vi "Joystick.vi"() -> ()   [LabVIEW 2020]
uses:
  <vilib>/Rock Robotics/WPI/Utilities/WPI_GetSetVariantRefNum.vi
  GlobalVariables.vi
  <vilib>/Rock Robotics/Network Tables/NT Write Number.vi
  <vilib>/Rock Robotics/WPI/RobotDrive/WPI_RobotDriveArcadeDrive_Standard(NoSaturation).vi
  <vilib>/Rock Robotics/WPI/ThirdParty/Phoenix-LabVIEW/Motor Controller/Controls/CTRE_Phoenix_MotorControl_ControlMode.ctl
panel:
  out "Hori":dbl
  out "Vert":dbl
  out "L_X":dbl
  out "L_Y":dbl
  out "Axes[3]":dbl
  out "Axes[2]":dbl
  out "Motor Values":dbl[](array[numeric])
  out "Axes[1]":dbl
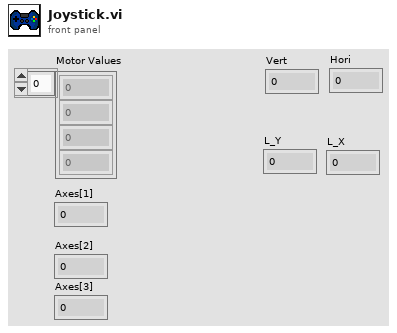
[diagram p1: front panel]
types:
  T1 = cluster{"Axes[0]":dbl, "Axes[1]":dbl, "Axes[2]":dbl, "Axes[3]":dbl, "Axes[4]":dbl, "Axes[5]":dbl, "Axes[6]":dbl, "Axes[7]":dbl, "Axes[8]":dbl}
  T2 = cluster{"Buttons[0]":bool, "Buttons[1]":bool, "Buttons[2]":bool, "Buttons[3]":bool, "Buttons[4]":bool, "Buttons[5]":bool, "Buttons[6]":bool, "Buttons[7]":bool, "Buttons[8]":bool, "Buttons[9]":bool}
  T3 = typedef "WPI_RobotDriveDevRef.ctl" = cluster{"DevStatus":errorcluster, "Motors[]":T4[], "Square Inputs":bool, "Max Output":dbl}
  T4 = typedef "WPI_MotorControlDeviceRef.ctl" = cluster{"DeviceStatus":errorcluster, "Type":T5, "PWM":cluster{"PWM Channel":T6, "DeadBand":T7}, "CAN":cluster{"Device Number":u8, "SetOutput VI Ref":variant, "GetOutput VI Ref":variant, "Enable VI Ref":variant, "Disable VI Ref":variant, "Data":variant}, "Invert":bool, "DIO PWM":cluster{"PWM \"Enable\" Channel":T6, "DIOChannel":T8, "PWM Rate":dbl}}
  T5 = typedef "WPI_MotorControlType.ctl" = enum16{"PWM", "CAN", "DIO PWM"}
  T6 = typedef "FPGA_DIOPWMChannel.ctl" = enum8{"PWM 0", "PWM 1", "PWM 2", "PWM 3", "PWM 4", "PWM 5", "PWM 6", "PWM 7", "PWM 8", "PWM 9", "PWM MXP 0", "PWM MXP 1", "PWM MXP 2", "PWM MXP 3", "PWM MXP 4", "PWM MXP 5", "PWM MXP 6", "PWM MXP 7", "PWM MXP 8", "PWM MXP 9", "Invalid"}
  T7 = typedef "WPI_PWMDeadband.ctl" = cluster{"Name":string, "maxPositivePwm":i32, "minPositivePwm":i32, "centerPwm":i32, "maxNegativePwm":i32, "minNegativePwm":i32, "angularRange":u16}
  T8 = typedef "FPGA_DIOChannel.ctl" = enum8{"DIO 0", "DIO 1", "DIO 2", "DIO 3", "DIO 4", "DIO 5", "DIO 6", "DIO 7", "DIO 8", "DIO 9", "DIO MXP 0", "DIO MXP 1", "DIO MXP 2", "DIO MXP 3", "DIO MXP 4", "DIO MXP 5", "DIO MXP 6", "DIO MXP 7", "DIO MXP 8", "DIO MXP 9", "DIO MXP 10", "DIO MXP 11", "DIO MXP 12", "DIO MXP 13", "DIO MXP 14", "DIO MXP 15", "SPI Port CS1", "SPI Port CS2", "SPI Port CS3", "SPI Port MISO", "SPI Port MOSI", "Invalid"}
  T9 = typedef "CTRE_Phoenix_MotorControl_ControlMode.ctl" = u16
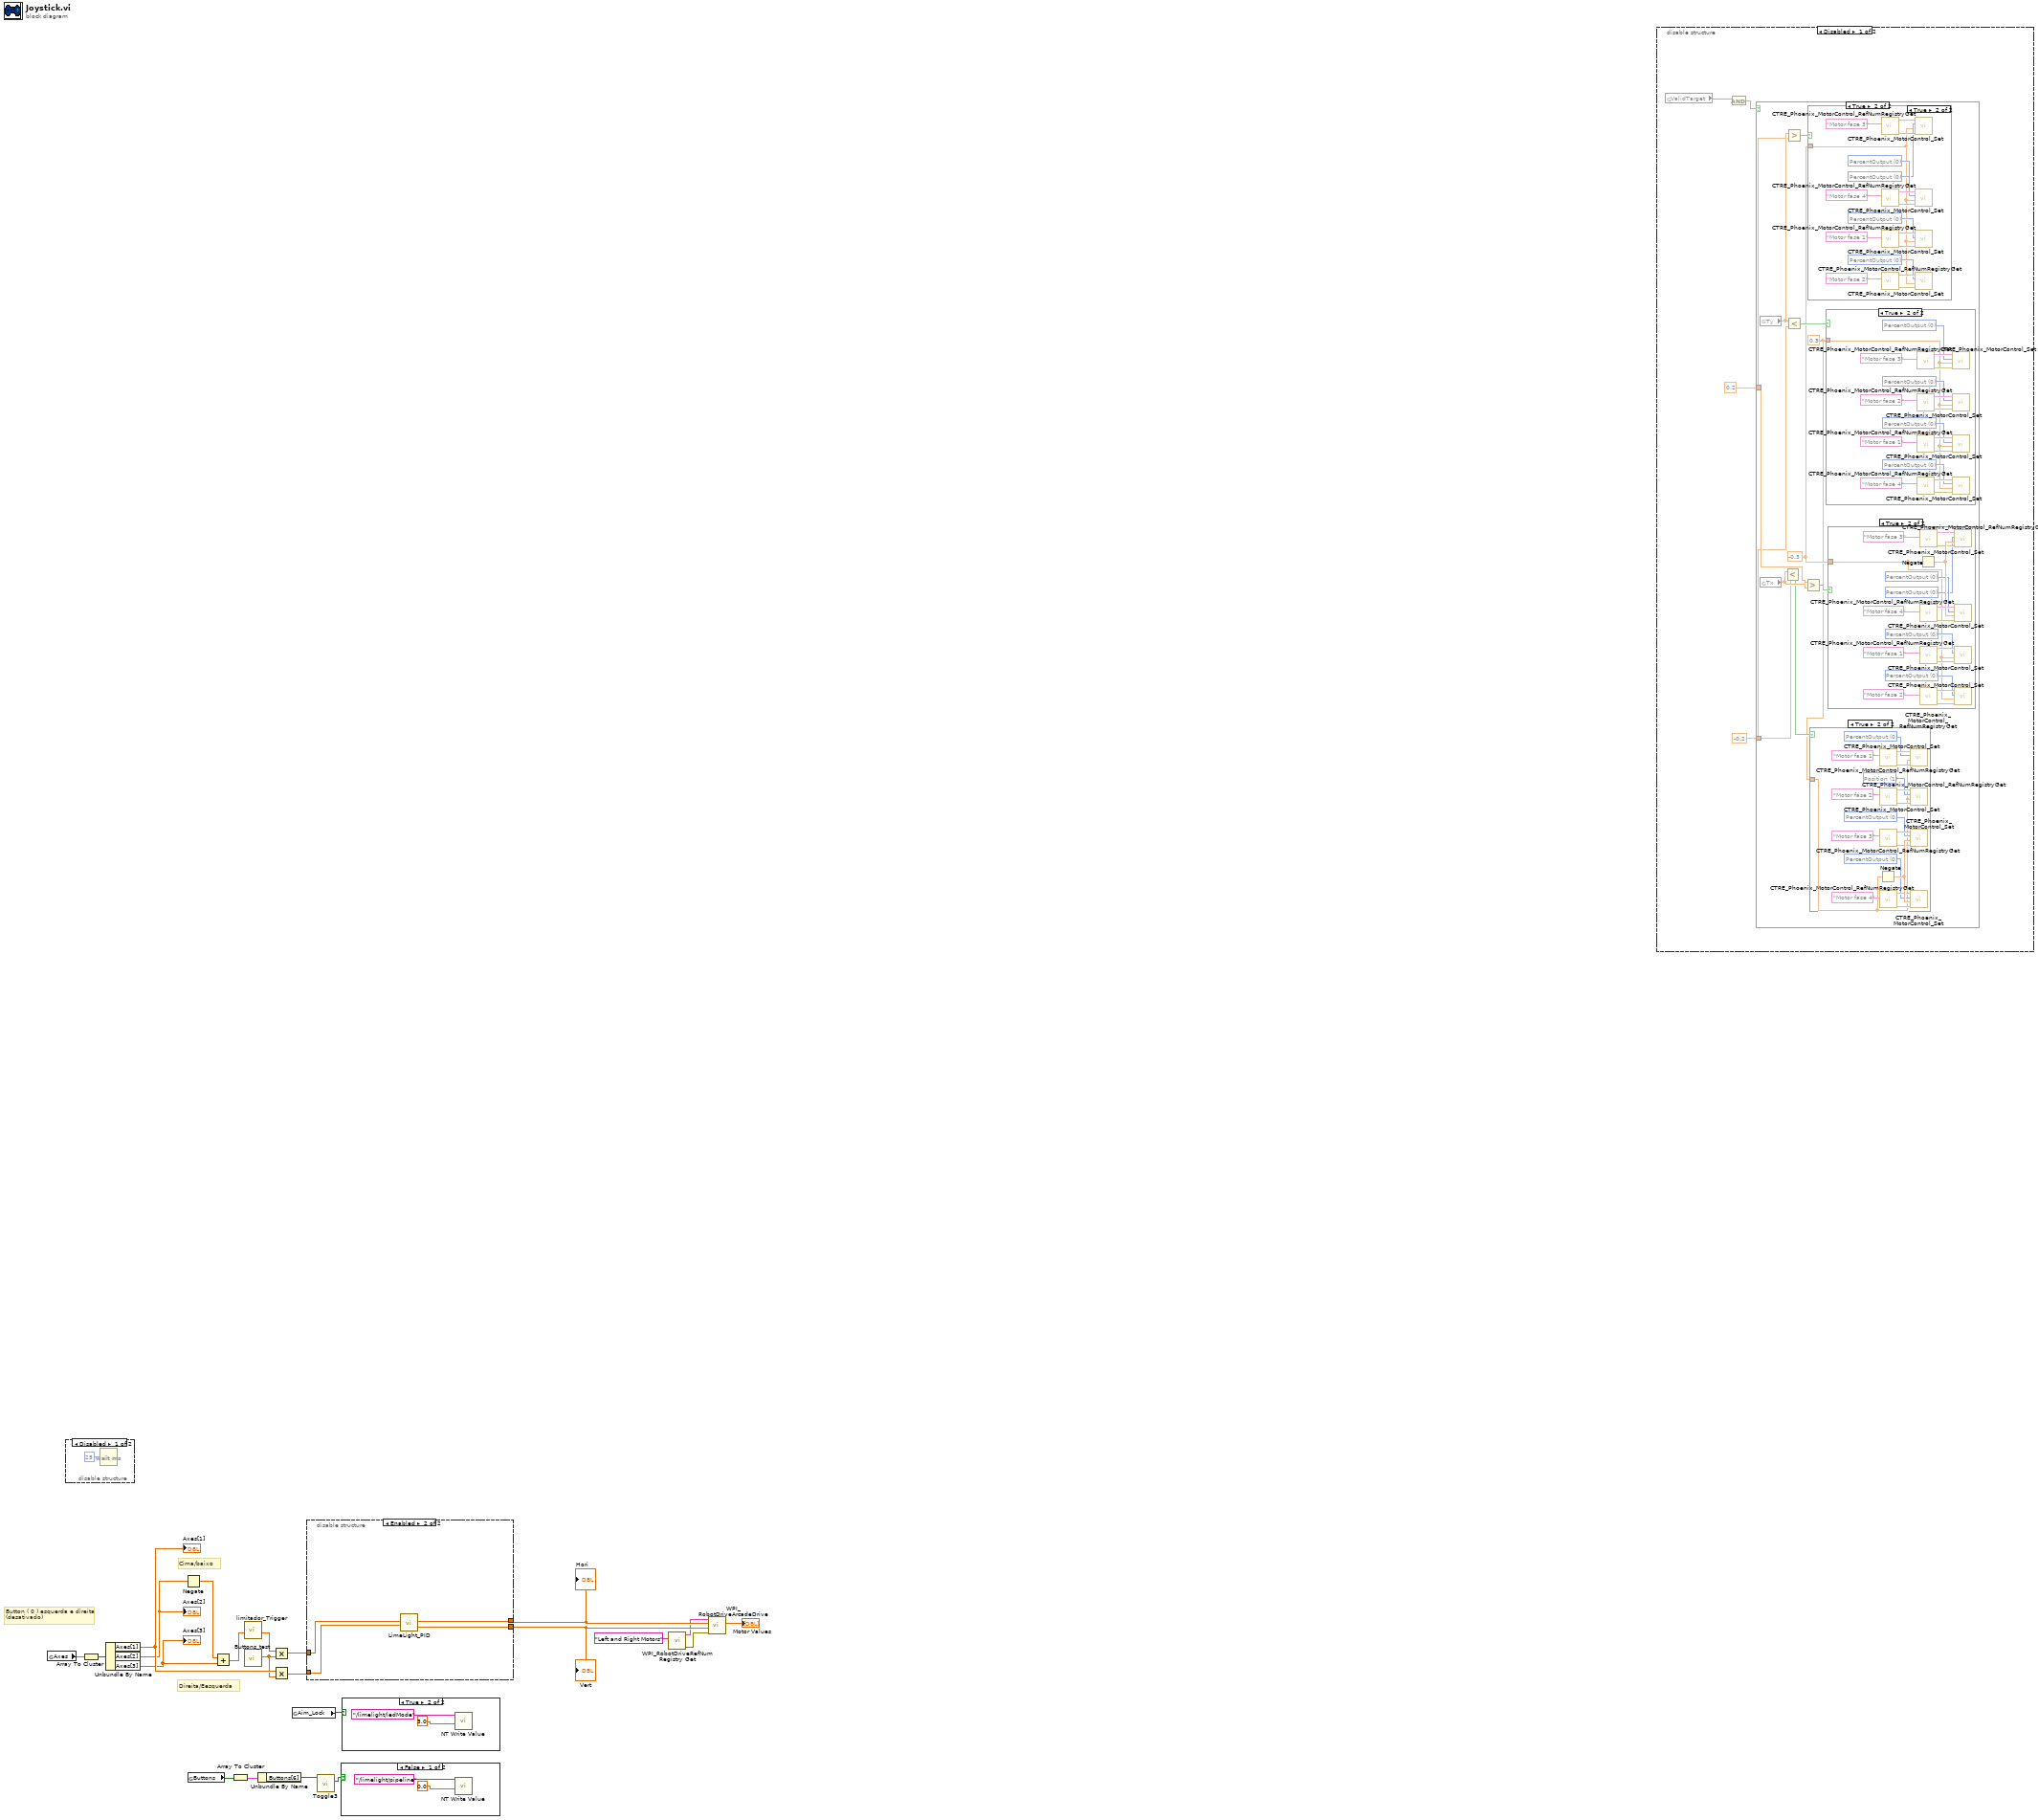
[diagram p0: block diagram]
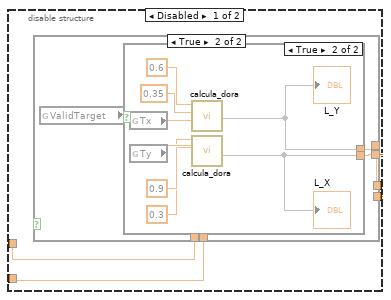
[diagram p3: hidden frame]
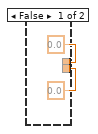
[diagram p5: hidden frame]
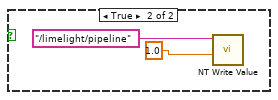
[diagram p6: hidden frame]
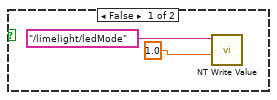
[diagram p7: hidden frame]
diagram:
  # "Button ( 0 ) esquerda e direita \n(desativado)"
  # "Direita/Eesquerda"
  # "Cima/baixo"
  n1 = global read "GlobalVariables.vi" "Axes"() -> (w3:dbl[])
  n2 = disable-structure shown="Disabled" {
    frame Disabled {
      n3 = Wait (ms)(milliseconds to wait=u32 25) -> ()  [unwired: 1 out]
    }
    frame Enabled {
    }
  }
  n4 = Array To Cluster(array=w3) -> (cluster=w4:T1)
  n5 = Unbundle By Name(w4) -> ("Axes[1]"=w22:dbl, "Axes[2]"=w18:dbl, "Axes[3]"=w7:dbl)
  "Axes[1]" <- w22
  "Axes[2]" <- w18
  "Axes[3]" <- w7
  n6 = Negate(x=w18) -> (-x=w17:dbl)
  n7 = global read "GlobalVariables.vi" "Buttons"() -> (w5:bool[])
  n8 = Add(x=w17, y=w7) -> (x+y=w20:dbl)
  n9 = Array To Cluster(array=w5) -> (cluster=w6:T2)
  n10 = call "limitador_Trigger.vi"("IN"=w20) -> ("OUT"=w19:dbl)  [unwired: 10 in]
  n11 = call "Buttons_test.vi"() -> ("OUT"=w21:dbl)  [unwired: 9 in]
  n12 = Unbundle By Name(w6) -> ("Buttons[6]"=w1:bool)
  n13 = Multiply(x=w19, y=w21) -> (x*y=w15:dbl)
  n14 = Multiply(x=w22, y=w21) -> (x*y=w16:dbl)
  n15 = global read "GlobalVariables.vi" "Aim_Lock"() -> (w8:bool)
  n16 = disable-structure shown="Enabled" {
    disable-tunnel: w16 -> [w27 w44]
    disable-tunnel: w15 -> [w26 w46]
    disable-tunnel: [w25 w45] -> w14
    disable-tunnel: [w24 w43] -> w13
    frame Disabled {
      n17 = case shown="True" {
        selector: _ -> [_ _]
        tunnel: w27 -> [w29 _]
        tunnel: w26 -> [w28 _]
        tunnel: [w29 w31] -> w25
        tunnel: [w28 w32] -> w24
        frame False {
        }
        frame True {
          n18 = global read "GlobalVariables.vi" "ValidTarget"() -> (w30:bool)
          n19 = case shown="True" w30 {
            tunnel: [0.0 ("x+y") w42] -> w32
            tunnel: [0.0 ("x+y") w39] -> w31
            frame False {
            }
            frame True {
              n20 = global read "GlobalVariables.vi" "Tx"() -> (w41:dbl)
              n21 = global read "GlobalVariables.vi" "Ty"() -> (w40:dbl)
              n22 = call "calcula_dora.vi"(9:w41, 10:0.35, 11:0.6) -> (1:w42)  [unwired: 8 in]
              "L_Y" <- w42
              n23 = call "calcula_dora.vi"(9:w40, 10:0.3, 11:0.9) -> (1:w39)  [unwired: 8 in]
              "L_X" <- w39
            }
          }
        }
      }
    }
    frame Enabled {
      n24 = call "LimeLight_PID.vi"("Numeric 2"=w44, "Numeric"=w46) -> ("output_ty"=w45:dbl, "output_tx"=w43:dbl)  [unwired: 8 in]
    }
  }
  "Vert" <- w14
  "Hori" <- w13
  n25 = call "Toggle3.vi"("Input3"=w1) -> ("Output3"=w2:bool)  [unwired: 10 in]
  n26 = case shown="False" w2 {
    frame False {
      n27 = call-poly <vilib>:"NT Write Value.vi"("Numeric"=0.0, "Name"="/limelight/pipeline") -> ()  [unwired: 9 in, 1 out]
    }
    frame True {
      n28 = call-poly <vilib>:"NT Write Value.vi"("Numeric"=1.0, "Name"="/limelight/pipeline") -> ()  [unwired: 9 in, 1 out]
    }
  }
  n29 = case shown="True" w8 {
    frame False {
      n30 = call-poly <vilib>:"NT Write Value.vi"("Numeric"=1.0, "Name"="/limelight/ledMode") -> ()  [unwired: 9 in, 1 out]
    }
    frame True {
      n31 = call-poly <vilib>:"NT Write Value.vi"("Numeric"=3.0, "Name"="/limelight/ledMode") -> ()  [unwired: 9 in, 1 out]
    }
  }
  n32 = call <vilib>:"WPI_RobotDriveRefNum Registry Get.vi"("refnum name"="Left and Right Motors") -> ("error out"=w9:errorcluster, "RobotDriveDevRef"=w11:T3)  [unwired: 9 in]
  n33 = call-poly <vilib>:"WPI_RobotDriveArcadeDrive.vi"("error in (no error)"=w9, "Y axis value"=w14, "X axis value"=w13, "RobotDriveDevRef"=w11) -> ("Motor Values"=→"Motor Values":dbl[])  [unwired: 5 in, 2 out]
  n34 = disable-structure shown="Disabled" {
    frame Disabled {
      n35 = global read "GlobalVariables.vi" "ValidTarget"() -> (w58:bool)
      n36 = And(x=w58) -> (x .and. y?=w57:bool)  [unwired: 1 in]
      n37 = case shown="True" w57 {
        tunnel: 0.2 -> [_ w62]
        tunnel: -0.2 -> [_ w61]
        frame False {
        }
        frame True {
          w59 = 0.3
          w60 = -0.3
          n38 = global read "GlobalVariables.vi" "Ty"() -> (w64:dbl)
          n39 = global read "GlobalVariables.vi" "Tx"() -> (w67:dbl)
          n40 = Less?(x=w67, y=w61) -> (x < y?=w66:bool)
          n41 = Greater?(x=w64, y=w62) -> (0:w65:bool)
          n42 = Less?(x=w64, y=w61) -> (x < y?=w63:bool)
          n43 = Greater?(x=w67, y=w62) -> (0:w68:bool)
          n44 = case shown="True" w65 {
            tunnel: w60 -> [_ w86]
            frame False {
            }
            frame True {
              w94 = T9 0 items=["PercentOutput"=0, "Position"=1, "Velocity"=2, "Current"=3, "Follower"=5, "MotionProfile"=6, "MotionMagic"=7, "MotionProfileArc"=10, "Disabled"=15] ("Control Mode")
              w92 = T9 0 items=["PercentOutput"=0, "Position"=1, "Velocity"=2, "Current"=3, "Follower"=5, "MotionProfile"=6, "MotionMagic"=7, "MotionProfileArc"=10, "Disabled"=15] ("Control Mode")
              w90 = T9 0 items=["PercentOutput"=0, "Position"=1, "Velocity"=2, "Current"=3, "Follower"=5, "MotionProfile"=6, "MotionMagic"=7, "MotionProfileArc"=10, "Disabled"=15] ("Control Mode")
              w88 = T9 0 items=["PercentOutput"=0, "Position"=1, "Velocity"=2, "Current"=3, "Follower"=5, "MotionProfile"=6, "MotionMagic"=7, "MotionProfileArc"=10, "Disabled"=15] ("Control Mode")
              n45 = call <vilib>:"CTRE_Phoenix_MotorControl_RefNumRegistryGet.vi"("refnum name"="Motor fase 3") -> ("error out"=w96:errorcluster, "PhoenixMotorControlDevRef"=w95:T4)  [unwired: 9 in]
              n46 = call <vilib>:"CTRE_Phoenix_MotorControl_RefNumRegistryGet.vi"("refnum name"="Motor fase 4") -> ("error out"=w98:errorcluster, "PhoenixMotorControlDevRef"=w97:T4)  [unwired: 9 in]
              n47 = call <vilib>:"CTRE_Phoenix_MotorControl_RefNumRegistryGet.vi"("refnum name"="Motor fase 1") -> ("error out"=w100:errorcluster, "PhoenixMotorControlDevRef"=w99:T4)  [unwired: 9 in]
              n48 = call <vilib>:"CTRE_Phoenix_MotorControl_RefNumRegistryGet.vi"("refnum name"="Motor fase 2") -> ("error out"=w102:errorcluster, "PhoenixMotorControlDevRef"=w101:T4)  [unwired: 9 in]
              n49 = call <vilib>:"CTRE_Phoenix_MotorControl_Set.vi"("error in (no error)"=w96, "Output"=w86, "Control Mode"=w88, "PhoenixMotorControlDevRef"=w95) -> ()  [unwired: 6 in, 2 out]
              n50 = call <vilib>:"CTRE_Phoenix_MotorControl_Set.vi"("error in (no error)"=w98, "Output"=w86, "Control Mode"=w90, "PhoenixMotorControlDevRef"=w97) -> ()  [unwired: 6 in, 2 out]
              n51 = call <vilib>:"CTRE_Phoenix_MotorControl_Set.vi"("error in (no error)"=w100, "Output"=w86, "Control Mode"=w92, "PhoenixMotorControlDevRef"=w99) -> ()  [unwired: 6 in, 2 out]
              n52 = call <vilib>:"CTRE_Phoenix_MotorControl_Set.vi"("error in (no error)"=w102, "Output"=w86, "Control Mode"=w94, "PhoenixMotorControlDevRef"=w101) -> ()  [unwired: 6 in, 2 out]
            }
          }
          n53 = case shown="True" w66 {
            tunnel: w59 -> [_ w103]
            frame False {
            }
            frame True {
              w111 = T9 0 items=["PercentOutput"=0, "Position"=1, "Velocity"=2, "Current"=3, "Follower"=5, "MotionProfile"=6, "MotionMagic"=7, "MotionProfileArc"=10, "Disabled"=15] ("Control Mode")
              w109 = T9 0 items=["PercentOutput"=0, "Position"=1, "Velocity"=2, "Current"=3, "Follower"=5, "MotionProfile"=6, "MotionMagic"=7, "MotionProfileArc"=10, "Disabled"=15] ("Control Mode")
              w107 = T9 1 items=["PercentOutput"=0, "Position"=1, "Velocity"=2, "Current"=3, "Follower"=5, "MotionProfile"=6, "MotionMagic"=7, "MotionProfileArc"=10, "Disabled"=15] ("Control Mode")
              w105 = T9 0 items=["PercentOutput"=0, "Position"=1, "Velocity"=2, "Current"=3, "Follower"=5, "MotionProfile"=6, "MotionMagic"=7, "MotionProfileArc"=10, "Disabled"=15] ("Control Mode")
              n54 = call <vilib>:"CTRE_Phoenix_MotorControl_RefNumRegistryGet.vi"("refnum name"="Motor fase 1") -> ("error out"=w113:errorcluster, "PhoenixMotorControlDevRef"=w112:T4)  [unwired: 9 in]
              n55 = call <vilib>:"CTRE_Phoenix_MotorControl_RefNumRegistryGet.vi"("refnum name"="Motor fase 2") -> ("error out"=w115:errorcluster, "PhoenixMotorControlDevRef"=w114:T4)  [unwired: 9 in]
              n56 = call <vilib>:"CTRE_Phoenix_MotorControl_RefNumRegistryGet.vi"("refnum name"="Motor fase 3") -> ("error out"=w117:errorcluster, "PhoenixMotorControlDevRef"=w116:T4)  [unwired: 9 in]
              n57 = Negate(x=w103) -> (-x=w120:dbl)
              n58 = call <vilib>:"CTRE_Phoenix_MotorControl_RefNumRegistryGet.vi"("refnum name"="Motor fase 4") -> ("error out"=w119:errorcluster, "PhoenixMotorControlDevRef"=w118:T4)  [unwired: 9 in]
              n59 = call <vilib>:"CTRE_Phoenix_MotorControl_Set.vi"("error in (no error)"=w113, "Output"=w103, "Control Mode"=w105, "PhoenixMotorControlDevRef"=w112) -> ()  [unwired: 6 in, 2 out]
              n60 = call <vilib>:"CTRE_Phoenix_MotorControl_Set.vi"("error in (no error)"=w115, "Output"=w103, "Control Mode"=w107, "PhoenixMotorControlDevRef"=w114) -> ()  [unwired: 6 in, 2 out]
              n61 = call <vilib>:"CTRE_Phoenix_MotorControl_Set.vi"("error in (no error)"=w117, "Output"=w120, "Control Mode"=w109, "PhoenixMotorControlDevRef"=w116) -> ()  [unwired: 6 in, 2 out]
              n62 = call <vilib>:"CTRE_Phoenix_MotorControl_Set.vi"("error in (no error)"=w119, "Output"=w120, "Control Mode"=w111, "PhoenixMotorControlDevRef"=w118) -> ()  [unwired: 6 in, 2 out]
            }
          }
          n63 = case shown="True" w63 {
            tunnel: w59 -> [_ w69]
            frame False {
            }
            frame True {
              w77 = T9 0 items=["PercentOutput"=0, "Position"=1, "Velocity"=2, "Current"=3, "Follower"=5, "MotionProfile"=6, "MotionMagic"=7, "MotionProfileArc"=10, "Disabled"=15] ("Control Mode")
              w75 = T9 0 items=["PercentOutput"=0, "Position"=1, "Velocity"=2, "Current"=3, "Follower"=5, "MotionProfile"=6, "MotionMagic"=7, "MotionProfileArc"=10, "Disabled"=15] ("Control Mode")
              w73 = T9 0 items=["PercentOutput"=0, "Position"=1, "Velocity"=2, "Current"=3, "Follower"=5, "MotionProfile"=6, "MotionMagic"=7, "MotionProfileArc"=10, "Disabled"=15] ("Control Mode")
              w71 = T9 0 items=["PercentOutput"=0, "Position"=1, "Velocity"=2, "Current"=3, "Follower"=5, "MotionProfile"=6, "MotionMagic"=7, "MotionProfileArc"=10, "Disabled"=15] ("Control Mode")
              n64 = call <vilib>:"CTRE_Phoenix_MotorControl_RefNumRegistryGet.vi"("refnum name"="Motor fase 3") -> ("error out"=w79:errorcluster, "PhoenixMotorControlDevRef"=w78:T4)  [unwired: 9 in]
              n65 = call <vilib>:"CTRE_Phoenix_MotorControl_RefNumRegistryGet.vi"("refnum name"="Motor fase 2") -> ("error out"=w85:errorcluster, "PhoenixMotorControlDevRef"=w84:T4)  [unwired: 9 in]
              n66 = call <vilib>:"CTRE_Phoenix_MotorControl_RefNumRegistryGet.vi"("refnum name"="Motor fase 1") -> ("error out"=w83:errorcluster, "PhoenixMotorControlDevRef"=w82:T4)  [unwired: 9 in]
              n67 = call <vilib>:"CTRE_Phoenix_MotorControl_RefNumRegistryGet.vi"("refnum name"="Motor fase 4") -> ("error out"=w81:errorcluster, "PhoenixMotorControlDevRef"=w80:T4)  [unwired: 9 in]
              n68 = call <vilib>:"CTRE_Phoenix_MotorControl_Set.vi"("error in (no error)"=w79, "Output"=w69, "Control Mode"=w71, "PhoenixMotorControlDevRef"=w78) -> ()  [unwired: 6 in, 2 out]
              n69 = call <vilib>:"CTRE_Phoenix_MotorControl_Set.vi"("error in (no error)"=w85, "Output"=w69, "Control Mode"=w77, "PhoenixMotorControlDevRef"=w84) -> ()  [unwired: 6 in, 2 out]
              n70 = call <vilib>:"CTRE_Phoenix_MotorControl_Set.vi"("error in (no error)"=w83, "Output"=w69, "Control Mode"=w75, "PhoenixMotorControlDevRef"=w82) -> ()  [unwired: 6 in, 2 out]
              n71 = call <vilib>:"CTRE_Phoenix_MotorControl_Set.vi"("error in (no error)"=w81, "Output"=w69, "Control Mode"=w73, "PhoenixMotorControlDevRef"=w80) -> ()  [unwired: 6 in, 2 out]
            }
          }
          n72 = case shown="True" w68 {
            tunnel: w60 -> [_ w121]
            frame False {
            }
            frame True {
              w129 = T9 0 items=["PercentOutput"=0, "Position"=1, "Velocity"=2, "Current"=3, "Follower"=5, "MotionProfile"=6, "MotionMagic"=7, "MotionProfileArc"=10, "Disabled"=15] ("Control Mode")
              w127 = T9 0 items=["PercentOutput"=0, "Position"=1, "Velocity"=2, "Current"=3, "Follower"=5, "MotionProfile"=6, "MotionMagic"=7, "MotionProfileArc"=10, "Disabled"=15] ("Control Mode")
              w125 = T9 0 items=["PercentOutput"=0, "Position"=1, "Velocity"=2, "Current"=3, "Follower"=5, "MotionProfile"=6, "MotionMagic"=7, "MotionProfileArc"=10, "Disabled"=15] ("Control Mode")
              w123 = T9 0 items=["PercentOutput"=0, "Position"=1, "Velocity"=2, "Current"=3, "Follower"=5, "MotionProfile"=6, "MotionMagic"=7, "MotionProfileArc"=10, "Disabled"=15] ("Control Mode")
              n73 = call <vilib>:"CTRE_Phoenix_MotorControl_RefNumRegistryGet.vi"("refnum name"="Motor fase 3") -> ("error out"=w135:errorcluster, "PhoenixMotorControlDevRef"=w134:T4)  [unwired: 9 in]
              n74 = Negate(x=w121) -> (-x=w138:dbl)
              n75 = call <vilib>:"CTRE_Phoenix_MotorControl_RefNumRegistryGet.vi"("refnum name"="Motor fase 4") -> ("error out"=w137:errorcluster, "PhoenixMotorControlDevRef"=w136:T4)  [unwired: 9 in]
              n76 = call <vilib>:"CTRE_Phoenix_MotorControl_RefNumRegistryGet.vi"("refnum name"="Motor fase 1") -> ("error out"=w131:errorcluster, "PhoenixMotorControlDevRef"=w130:T4)  [unwired: 9 in]
              n77 = call <vilib>:"CTRE_Phoenix_MotorControl_RefNumRegistryGet.vi"("refnum name"="Motor fase 2") -> ("error out"=w133:errorcluster, "PhoenixMotorControlDevRef"=w132:T4)  [unwired: 9 in]
              n78 = call <vilib>:"CTRE_Phoenix_MotorControl_Set.vi"("error in (no error)"=w135, "Output"=w138, "Control Mode"=w127, "PhoenixMotorControlDevRef"=w134) -> ()  [unwired: 6 in, 2 out]
              n79 = call <vilib>:"CTRE_Phoenix_MotorControl_Set.vi"("error in (no error)"=w137, "Output"=w138, "Control Mode"=w129, "PhoenixMotorControlDevRef"=w136) -> ()  [unwired: 6 in, 2 out]
              n80 = call <vilib>:"CTRE_Phoenix_MotorControl_Set.vi"("error in (no error)"=w131, "Output"=w121, "Control Mode"=w123, "PhoenixMotorControlDevRef"=w130) -> ()  [unwired: 6 in, 2 out]
              n81 = call <vilib>:"CTRE_Phoenix_MotorControl_Set.vi"("error in (no error)"=w133, "Output"=w121, "Control Mode"=w125, "PhoenixMotorControlDevRef"=w132) -> ()  [unwired: 6 in, 2 out]
            }
          }
        }
      }
    }
    frame Enabled {
    }
  }
